vi "arrayBoolean.vi"(1 "Array In":bool[](array[boolean])) -> (0 "Array Out":bool[](array[boolean]))   [LabVIEW 2012]
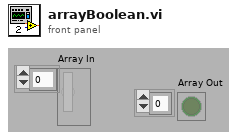
[diagram p1: front panel]
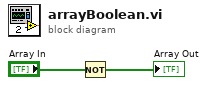
[diagram p0: block diagram]
diagram:
  n1 = Not(x="Array In") -> (.not. x?=→"Array Out":bool[])
